vi "Convert View Arrays to 3x3.vi"(4 "Values":i32[](array[numeric]), 5 "Directions":T1[](array[typedef])) -> (1 "I32 3x3 Grid Out":T2)   [LabVIEW 2017, in "AntFarm_MB.lvclass"]
uses:
  AntFarm_MB.lvclass
  TypeDefs/Cluster_I32 3x3 Grid.ctl
  Type Defs/Direction Enum.ctl
  Type Defs/SB Type Defs.lvlib
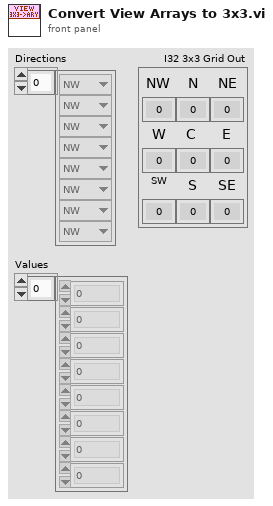
[diagram p1: front panel]
types:
  T1 = typedef "SB Type Defs.lvlib/Direction Enum.ctl" = enum16{"NW", "N", "NE", "E", "SE", "S", "SW", "W"}
  T2 = typedef "Cluster_I32 3x3 Grid.ctl" = cluster{"NW":i32, "N":i32, "NE":i32, "E":i32, "SE":i32, "S":i32, "SW":i32, "W":i32, "C":i32}
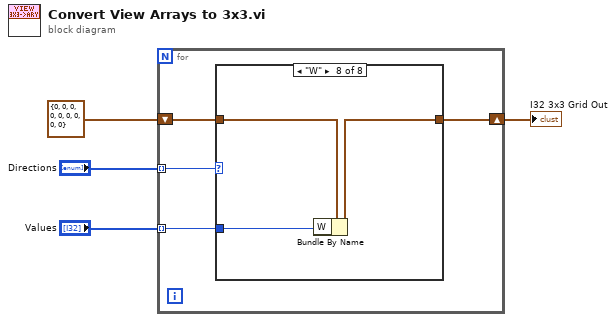
[diagram p0: block diagram]
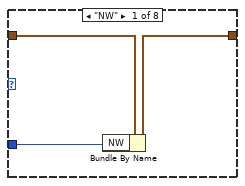
[diagram p2: hidden frame]
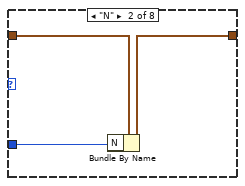
[diagram p3: hidden frame]
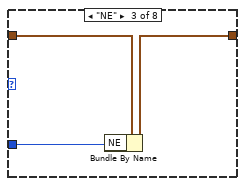
[diagram p4: hidden frame]
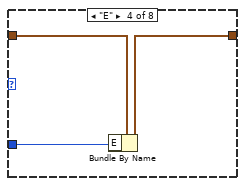
[diagram p5: hidden frame]
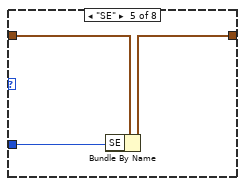
[diagram p6: hidden frame]
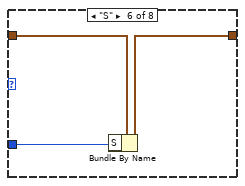
[diagram p7: hidden frame]
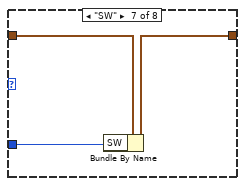
[diagram p8: hidden frame]
diagram:
  n1 = for {
    shift-right: [w6] -> w3
    shift-left: T2 {"NW"=0, "N"=0, "NE"=0, "E"=0, "SE"=0, "S"=0, "SW"=0, "W"=0, "C"=0} ("I32 3x3 Grid") -> [w7]
    tunnel: "Directions" -> [w8] mode=indexing
    tunnel: "Values" -> [w5] mode=indexing
    n2 = case shown="\"W\"" w8 {
      tunnel: w7 -> [w11 w14 w17 w20 w23 w26 w29 w32]
      tunnel: [w10 w13 w16 w19 w22 w25 w28 w31] -> w6
      tunnel: w5 -> [w9 w12 w15 w18 w21 w24 w27 w30]
      frame "NW" {
        n3 = Bundle By Name(cluster=w11, "NW"=w9) -> (w10:T2)
      }
      frame "N" {
        n4 = Bundle By Name(cluster=w14, "N"=w12) -> (w13:T2)
      }
      frame "NE" {
        n5 = Bundle By Name(cluster=w17, "NE"=w15) -> (w16:T2)
      }
      frame "E" {
        n6 = Bundle By Name(cluster=w20, "E"=w18) -> (w19:T2)
      }
      frame "SE" {
        n7 = Bundle By Name(cluster=w23, "SE"=w21) -> (w22:T2)
      }
      frame "S" {
        n8 = Bundle By Name(cluster=w26, "S"=w24) -> (w25:T2)
      }
      frame "SW" {
        n9 = Bundle By Name(cluster=w29, "SW"=w27) -> (w28:T2)
      }
      frame "W" {
        n10 = Bundle By Name(cluster=w32, "W"=w30) -> (w31:T2)
      }
    }
  }
  "I32 3x3 Grid Out" <- w3
